vi "Alicat_command case v2.vi"(7 "Case":T1(ring), 8 "error in (no error)":errorcluster, 9 "Val 2":string, 10 "Val 1":i32, 11 "VISA resource name":refnum<visa-resource-name>) -> (0 "error out":errorcluster, 1 "bytes at port":u32, 2 "String From Alicat":string, 3 "dup VISA resource name":refnum<visa-resource-name>)   [LabVIEW 2016]
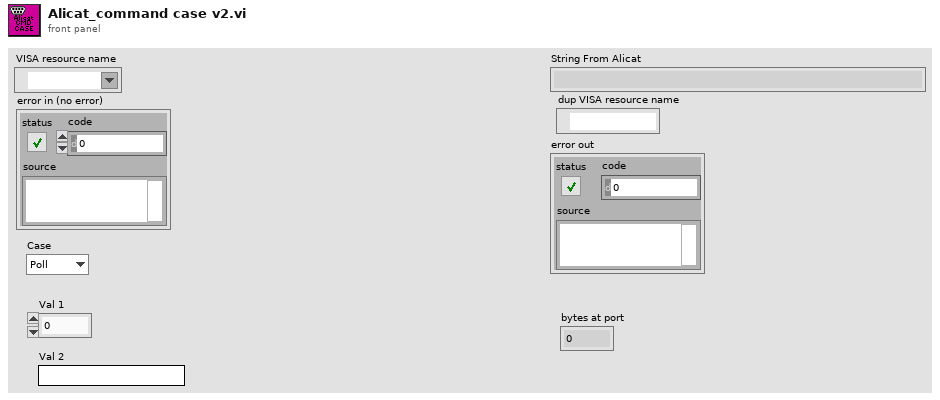
[diagram p1: front panel]
types:
  T1 = enum16{"Poll", "Set Stream", "Set Poll", "Define Set Point", "Gas Select", "Set P Gain", "Set D Gain", "Get P Gain", "Get D Gain", "Assign New Addess", ""}
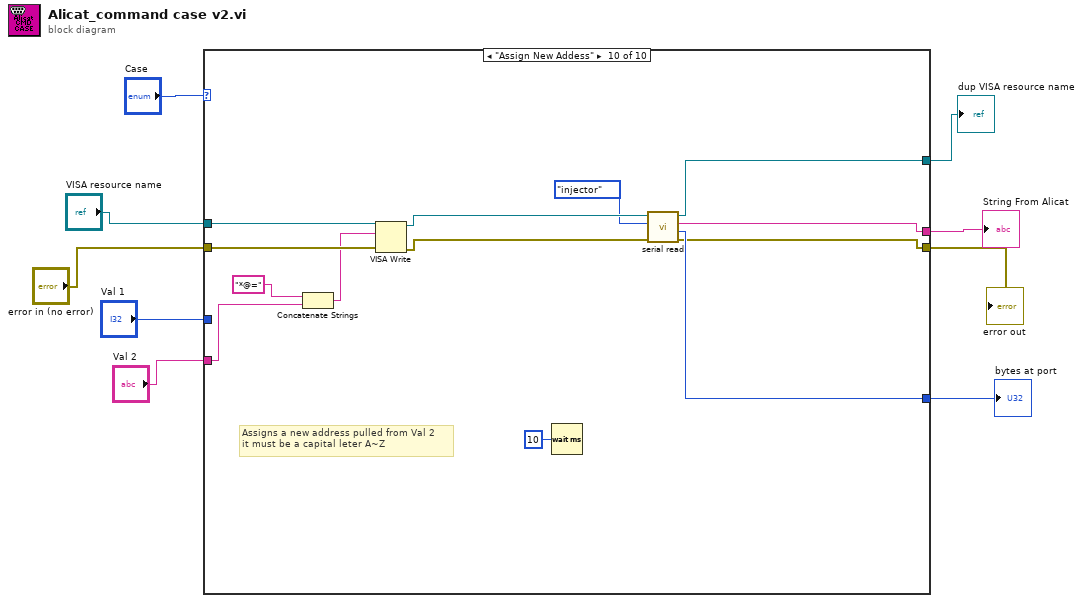
[diagram p0: block diagram]
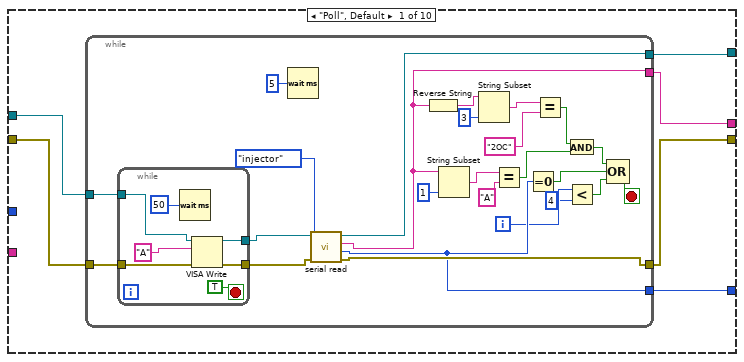
[diagram p2: hidden frame]
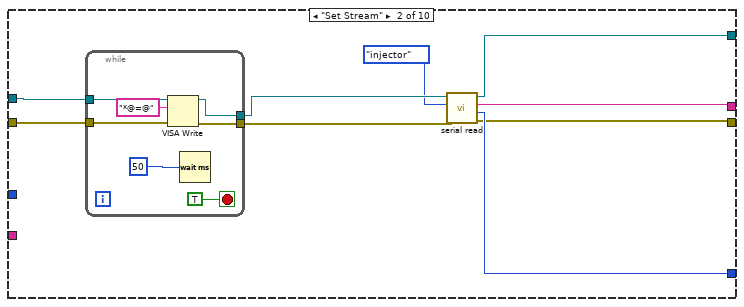
[diagram p3: hidden frame]
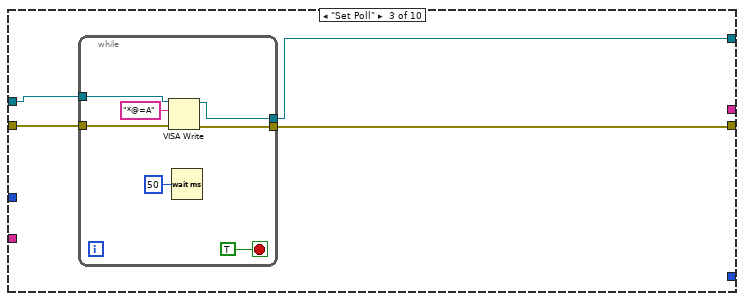
[diagram p4: hidden frame]
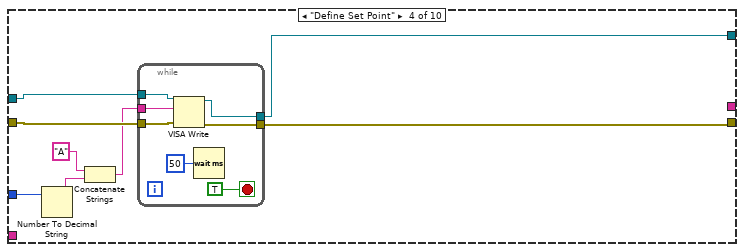
[diagram p5: hidden frame]
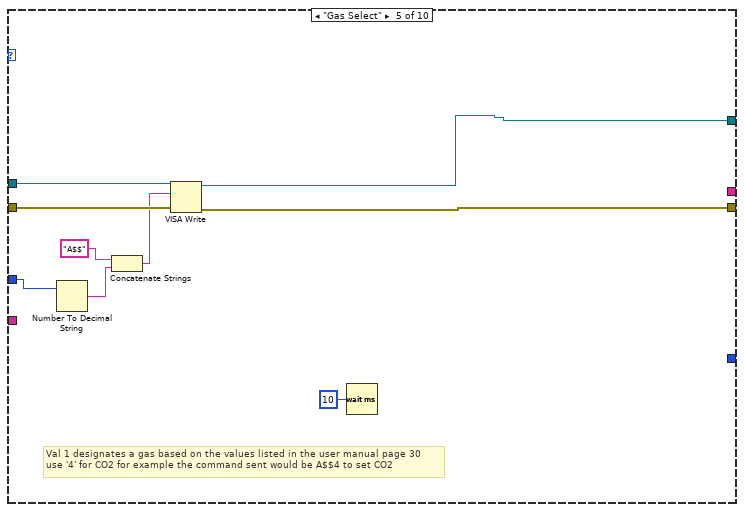
[diagram p6: hidden frame]
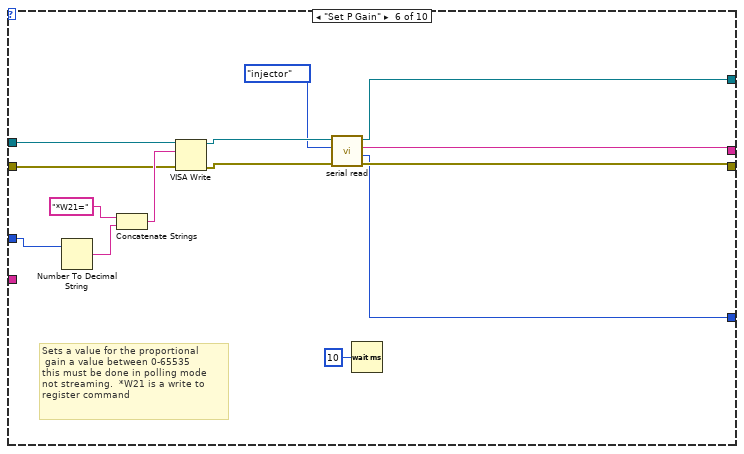
[diagram p7: hidden frame]
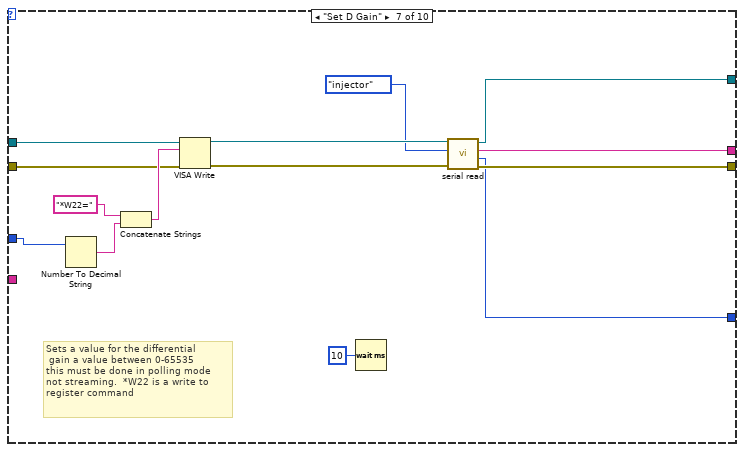
[diagram p8: hidden frame]
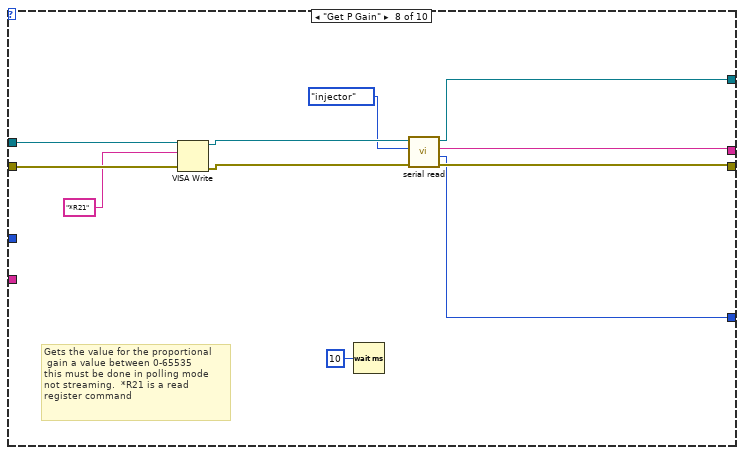
[diagram p9: hidden frame]
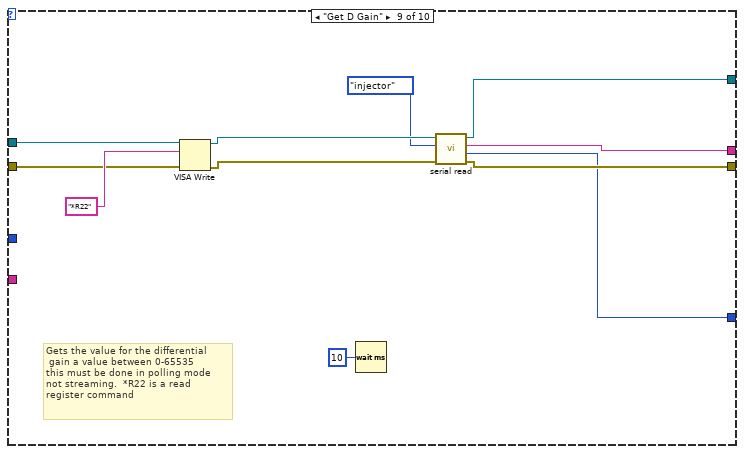
[diagram p10: hidden frame]
diagram:
  n1 = case shown="\"Assign New Addess\"" "Case" {
    tunnel: "VISA resource name" -> [w15 w56 w67 w82 w97 w108 w122 w136 w146 w160]
    tunnel: "error in (no error)" -> [w14 w55 w66 w81 w96 w107 w121 w135 w145 w159]
    tunnel: [w11 w52 w65 w76 w91 w100 w114 w128 w139 w153] -> w6
    tunnel: [w10 w49 w64 w75 w90 w103 w117 w131 w142 w150] -> w5
    tunnel: [w13 w51 _ _ _ w101 w115 w129 w140 w152] -> w7
    tunnel: "Val 2" -> [_ _ _ _ _ _ _ _ _ w158]
    tunnel: "Val 1" -> [_ _ _ w79 w95 w106 w120 _ _ _]
    tunnel: [w12 w50 _ _ _ w102 w116 w130 w141 w151] -> w1
    frame "Poll", Default {
      n2 = while {
        tunnel: [w35] -> w11
        tunnel: [w34] -> w10
        tunnel: w15 -> [w40]
        tunnel: w14 -> [w39]
        tunnel: [w26] -> w13
        tunnel: [w31] -> w12
        i -> [w17]
        stop <- w33 stop-if-true
        n3 = while {
          tunnel: w40 -> [w47]
          tunnel: w39 -> [w46]
          tunnel: [w45] -> w37
          tunnel: [w44] -> w36
          stop <- TRUE stop-if-true
          n4 = Wait (ms)(milliseconds to wait=u32 50) -> ()  [unwired: 1 out]
          n5 = VISA Write(VISA resource name=w47, write buffer="A", error in (no error)=w46) -> (VISA resource name out=w45:refnum<visa-resource-name>, error out=w44:errorcluster)  [unwired: 1 out]
        }
        n6 = Wait (ms)(milliseconds to wait=u32 5) -> ()  [unwired: 1 out]
        n7 = call "serial read.vi"("error in (no error)"=w36, "opMode"=enum16{"default", "injector", "gas analyzer"}."injector", "VISA resource name in"=w37) -> ("error out"=w34:errorcluster, "bytes count"=w31:u32, "read buffer"=w26:string, "VISA resource name out"=w35:refnum<visa-resource-name>)  [unwired: 5 in]
        n8 = Reverse String(1:w26) -> (0:w25:string)
        n9 = String Subset(string=w26, length (rest)=1 ("length (rest)")) -> (substring=w28:string)  [unwired: 1 in]
        n10 = String Subset(string=w25, length (rest)=3 ("length (rest)")) -> (substring=w23:string)  [unwired: 1 in]
        n11 = Equal?(x=w28, y="A") -> (x = y?=w20:bool)
        n12 = Equal To 0?(x=w31) -> (x = 0?=w32:bool)
        n13 = Equal?(x=w23, y="2OC" ("search string")) -> (x = y?=w21:bool)
        n14 = And(x=w21, y=w20) -> (x .and. y?=w19:bool)
        n15 = Less?(x=w17, y=4) -> (x < y?=w18:bool)
        n16 = Compound Arithmetic op=OR(w19, w32, w18) -> (w33:bool)
      }
    }
    frame "Set Stream" {
      n17 = while {
        tunnel: w56 -> [w62]
        tunnel: w55 -> [w61]
        tunnel: [w60] -> w54
        tunnel: [w59] -> w53
        stop <- TRUE stop-if-true
        n18 = VISA Write(VISA resource name=w62, write buffer="*@=@", error in (no error)=w61) -> (VISA resource name out=w60:refnum<visa-resource-name>, error out=w59:errorcluster)  [unwired: 1 out]
        n19 = Wait (ms)(milliseconds to wait=u32 50) -> ()  [unwired: 1 out]
      }
      n20 = call "serial read.vi"("error in (no error)"=w53, "opMode"=enum16{"default", "injector", "gas analyzer"}."injector", "VISA resource name in"=w54) -> ("error out"=w49:errorcluster, "bytes count"=w50:u32, "read buffer"=w51:string, "VISA resource name out"=w52:refnum<visa-resource-name>)  [unwired: 5 in]
    }
    frame "Set Poll" {
      n21 = while {
        tunnel: [w74] -> w65
        tunnel: [w73] -> w64
        tunnel: w67 -> [w71]
        tunnel: w66 -> [w70]
        stop <- TRUE stop-if-true
        n22 = VISA Write(VISA resource name=w71, write buffer="*@=A", error in (no error)=w70) -> (VISA resource name out=w74:refnum<visa-resource-name>, error out=w73:errorcluster)  [unwired: 1 out]
        n23 = Wait (ms)(milliseconds to wait=u32 50) -> ()  [unwired: 1 out]
      }
    }
    frame "Define Set Point" {
      n24 = Number To Decimal String(number=w79) -> (decimal integer string=w77:string)  [unwired: 1 in]
      n25 = Concatenate Strings("A" ("write buffer"), w77) -> (w78:string)
      n26 = while {
        tunnel: [w88] -> w76
        tunnel: [w87] -> w75
        tunnel: w82 -> [w86]
        tunnel: w81 -> [w85]
        tunnel: w78 -> [w84]
        stop <- TRUE stop-if-true
        n27 = VISA Write(VISA resource name=w86, write buffer=w84, error in (no error)=w85) -> (VISA resource name out=w88:refnum<visa-resource-name>, error out=w87:errorcluster)  [unwired: 1 out]
        n28 = Wait (ms)(milliseconds to wait=u32 50) -> ()  [unwired: 1 out]
      }
    }
    frame "Gas Select" {
      # "Val 1 designates a gas based on the values listed in the user manual page 30\nuse '4' for CO2 for example the command sent would be A$$4 to set CO2"
      n29 = Number To Decimal String(number=w95) -> (decimal integer string=w93:string)  [unwired: 1 in]
      n30 = Concatenate Strings("A$$" ("write buffer"), w93) -> (w92:string)
      n31 = VISA Write(VISA resource name=w97, write buffer=w92, error in (no error)=w96) -> (VISA resource name out=w91:refnum<visa-resource-name>, error out=w90:errorcluster)  [unwired: 1 out]
      n32 = Wait (ms)(milliseconds to wait=u32 10) -> ()  [unwired: 1 out]
    }
    frame "Set P Gain" {
      # "Sets a value for the proportional\n gain a value between 0-65535 \nthis must be done in polling mode \nnot streaming.  *W21 is a write to \nregister command"
      n33 = Number To Decimal String(number=w106) -> (decimal integer string=w110:string)  [unwired: 1 in]
      n34 = Concatenate Strings("*W21=" ("write buffer"), w110) -> (w109:string)
      n35 = VISA Write(VISA resource name=w108, write buffer=w109, error in (no error)=w107) -> (VISA resource name out=w105:refnum<visa-resource-name>, error out=w104:errorcluster)  [unwired: 1 out]
      n36 = call "serial read.vi"("error in (no error)"=w104, "opMode"=enum16{"default", "injector", "gas analyzer"}."injector", "VISA resource name in"=w105) -> ("error out"=w103:errorcluster, "bytes count"=w102:u32, "read buffer"=w101:string, "VISA resource name out"=w100:refnum<visa-resource-name>)  [unwired: 5 in]
      n37 = Wait (ms)(milliseconds to wait=u32 10) -> ()  [unwired: 1 out]
    }
    frame "Set D Gain" {
      # "Sets a value for the differential\n gain a value between 0-65535 \nthis must be done in polling mode \nnot streaming.  *W22 is a write to \nregister command"
      n38 = Number To Decimal String(number=w120) -> (decimal integer string=w124:string)  [unwired: 1 in]
      n39 = Concatenate Strings("*W22=" ("write buffer"), w124) -> (w123:string)
      n40 = VISA Write(VISA resource name=w122, write buffer=w123, error in (no error)=w121) -> (VISA resource name out=w119:refnum<visa-resource-name>, error out=w118:errorcluster)  [unwired: 1 out]
      n41 = Wait (ms)(milliseconds to wait=u32 10) -> ()  [unwired: 1 out]
      n42 = call "serial read.vi"("error in (no error)"=w118, "opMode"=enum16{"default", "injector", "gas analyzer"}."injector", "VISA resource name in"=w119) -> ("error out"=w117:errorcluster, "bytes count"=w116:u32, "read buffer"=w115:string, "VISA resource name out"=w114:refnum<visa-resource-name>)  [unwired: 5 in]
    }
    frame "Get P Gain" {
      # "Gets the value for the proportional\n gain a value between 0-65535 \nthis must be done in polling mode \nnot streaming.  *R21 is a read \nregister command"
      n43 = VISA Write(VISA resource name=w136, write buffer="*R21", error in (no error)=w135) -> (VISA resource name out=w133:refnum<visa-resource-name>, error out=w132:errorcluster)  [unwired: 1 out]
      n44 = Wait (ms)(milliseconds to wait=u32 10) -> ()  [unwired: 1 out]
      n45 = call "serial read.vi"("error in (no error)"=w132, "opMode"=enum16{"default", "injector", "gas analyzer"}."injector", "VISA resource name in"=w133) -> ("error out"=w131:errorcluster, "bytes count"=w130:u32, "read buffer"=w129:string, "VISA resource name out"=w128:refnum<visa-resource-name>)  [unwired: 5 in]
    }
    frame "Get D Gain" {
      # "Gets the value for the differential\n gain a value between 0-65535 \nthis must be done in polling mode \nnot streaming.  *R22 is a read \nregister command"
      n46 = VISA Write(VISA resource name=w146, write buffer="*R22", error in (no error)=w145) -> (VISA resource name out=w144:refnum<visa-resource-name>, error out=w143:errorcluster)  [unwired: 1 out]
      n47 = Wait (ms)(milliseconds to wait=u32 10) -> ()  [unwired: 1 out]
      n48 = call "serial read.vi"("error in (no error)"=w143, "opMode"=enum16{"default", "injector", "gas analyzer"}."injector", "VISA resource name in"=w144) -> ("error out"=w142:errorcluster, "bytes count"=w141:u32, "read buffer"=w140:string, "VISA resource name out"=w139:refnum<visa-resource-name>)  [unwired: 5 in]
    }
    frame "Assign New Addess" {
      # "Assigns a new address pulled from Val 2\nit must be a capital leter A~Z"
      n49 = Concatenate Strings("*@=" ("write buffer"), w158) -> (w156:string)
      n50 = VISA Write(VISA resource name=w160, write buffer=w156, error in (no error)=w159) -> (VISA resource name out=w155:refnum<visa-resource-name>, error out=w154:errorcluster)  [unwired: 1 out]
      n51 = Wait (ms)(milliseconds to wait=u32 10) -> ()  [unwired: 1 out]
      n52 = call "serial read.vi"("error in (no error)"=w154, "opMode"=enum16{"default", "injector", "gas analyzer"}."injector", "VISA resource name in"=w155) -> ("error out"=w150:errorcluster, "bytes count"=w151:u32, "read buffer"=w152:string, "VISA resource name out"=w153:refnum<visa-resource-name>)  [unwired: 5 in]
    }
  }
  "String From Alicat" <- w7
  "error out" <- w5
  "dup VISA resource name" <- w6
  "bytes at port" <- w1
